vi "Memory.Array.Initialize.vi"(8 "error in (no error)":errorcluster, 11 "Array in":refnum<class "Memory.Array.Void.lvclass">) -> (0 "error out":errorcluster, 3 "Array out":refnum<class "Memory.Array.Void.lvclass">)   [LabVIEW 2016, in "LabVIEW Memory Manager.lvlib" / "Memory.Array.Void.lvclass"]
uses:
  Memory.Array.Void.lvclass
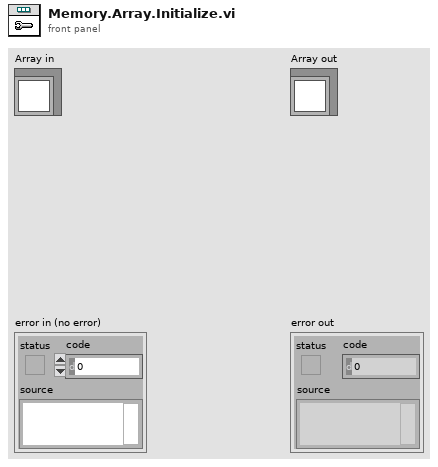
[diagram p1: front panel]
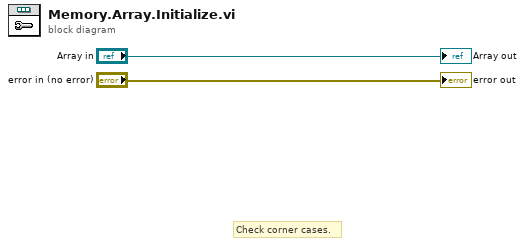
[diagram p0: block diagram]
diagram:
  # "Check corner cases."
  "error out" <- "error in (no error)"
  "Array out" <- "Array in"
